vi "CSM - Send Message and Wait for Reply.vi"(6 "Response Timeout(5000ms)":i32=5000, 7 "Current Module(\"\" to generate a ID)":string, 8 "Error In (no error)":errorcluster, 9 "Target Module":string="Target", 10 "Arguments (\"\")":string, 11 "State":string="API State") -> (0 "error out":errorcluster, 2 "Response":string="DoA", 4 ">> Source CSM >>":string)   [LabVIEW 2020, in "Communicable State Machine.lvlib"]
doc: "Send a message to CSM specified and wait for the reply with timeout.\n\n<b>Inputs:</b>\n - <b>Target Module</b>: Target CSM Module name.\n - <b>State</b>: Message to send\n - <b>Arguments (\"\")</b>: Argument of the message.\n - <b>Response Timeout(5000ms)</b>: Timeout for waiting the response.\n - <b>Error In (no error)</b>: Error cluster\n\n<b>Outputs:</b>\n - <b>Arguments</b>: Response returned.\n - <b>error out</b>: Error cluster"
uses:
  Communicable State Machine.lvlib
  Priority Queue.lvclass/Priority Queue.ctl
  _CSMObj-Message Check.vi
  _CSMObj-Enqueue Cross-Module Message.vi
  _CSMOFGV Get.vi
  Enqueue Element.vi
  _CSMOFGV.vi
  CSM Not Allowed Message.vi
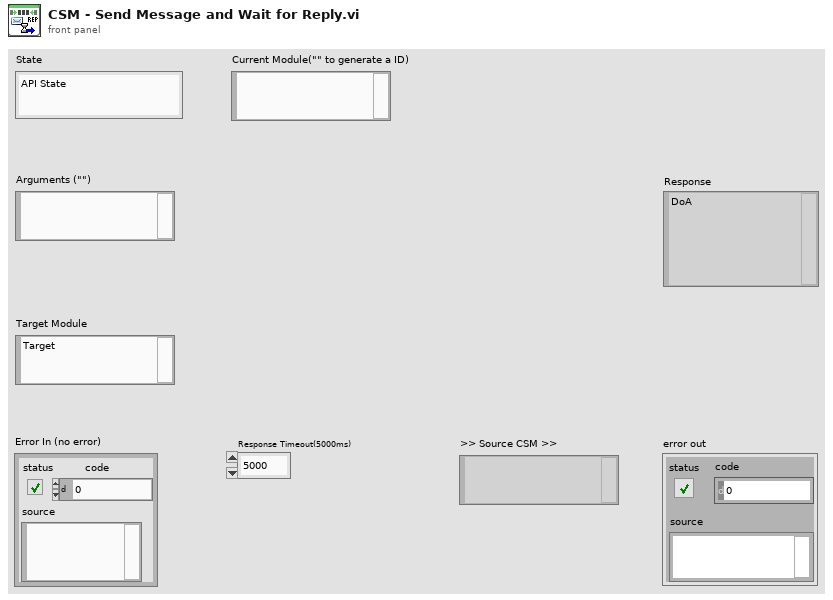
[diagram p1: front panel]
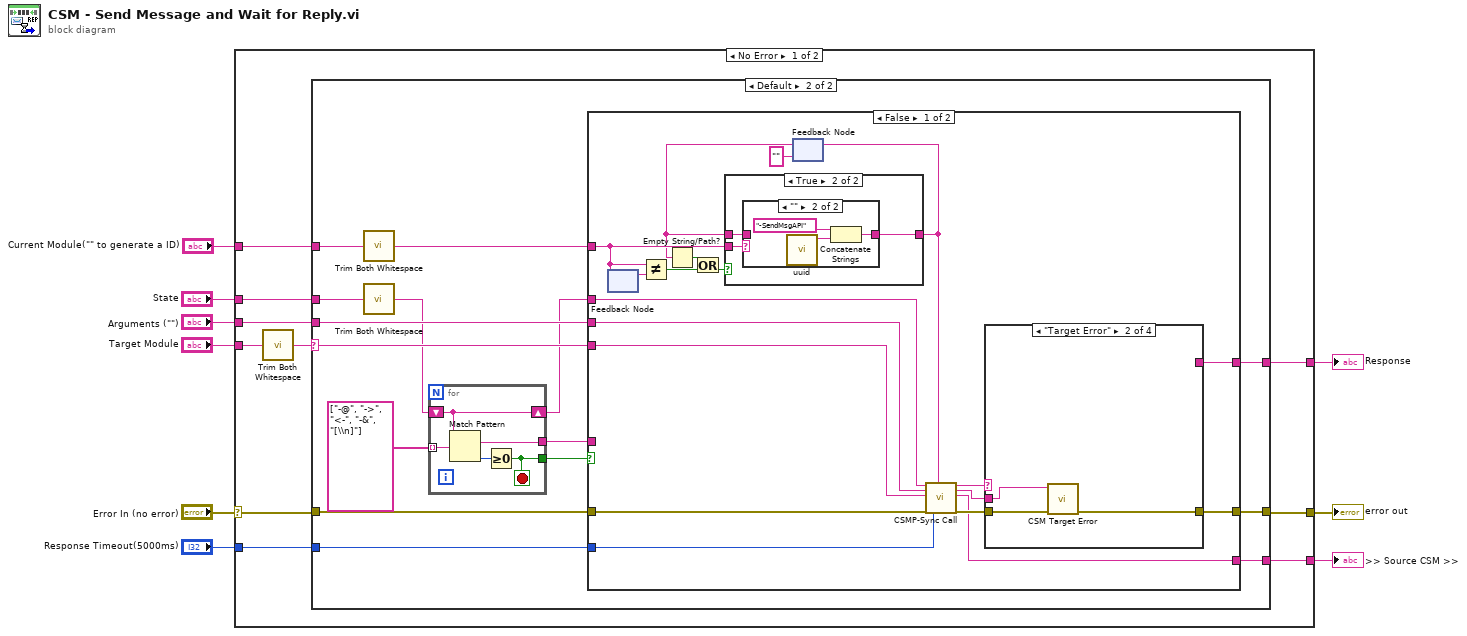
[diagram p0: block diagram]
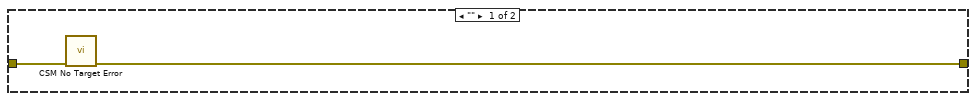
[diagram p2: hidden frame]
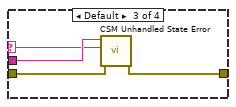
[diagram p6: hidden frame]
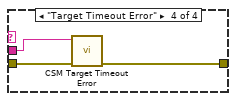
[diagram p7: hidden frame]
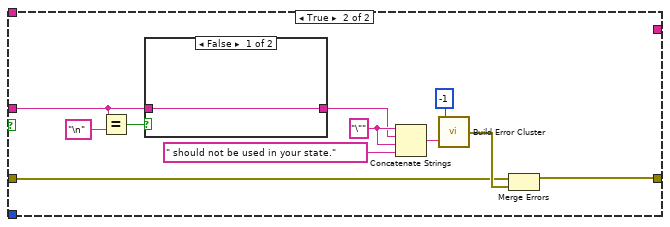
[diagram p8: hidden frame]
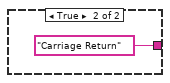
[diagram p9: hidden frame]
diagram:
  n1 = case shown="No Error" "Error In (no error)" {
    selector: "Error In (no error)" -> [w18 w94]
    tunnel: "State" -> [w19 _]
    tunnel: "Response Timeout(5000ms)" -> [w17 _]
    tunnel: [w13 w94] -> w6
    tunnel: [w16 _] -> w5
    tunnel: "Target Module" -> [w15 _]
    tunnel: "Arguments (\"\")" -> [w14 _]
    tunnel: "Current Module(\"\" to generate a ID)" -> [w11 _]
    tunnel: [w10 _] -> w1
    frame No Error {
      n2 = call "Trim Both Whitespace.vi"("string"=w15) -> ("trimmed string"=w12:string)  [unwired: 1 in]
      n3 = case shown="Default" w12 {
        selector: w12 -> [_ w33]
        tunnel: w18 -> [w21 w36]
        tunnel: w17 -> [_ w35]
        tunnel: [_ w34] -> w16
        tunnel: w14 -> [_ w32]
        tunnel: [w20 w31] -> w13
        tunnel: w19 -> [_ w30]
        tunnel: w11 -> [_ w23]
        tunnel: [_ w25] -> w10
        frame "" {
          n4 = call "CSM No Target Error.vi"("error in (no error)"=w21) -> ("error out"=w20:errorcluster)  [unwired: 10 in]
        }
        frame Default {
          n5 = call "Trim Both Whitespace.vi"("string"=w23) -> ("trimmed string"=w22:string)  [unwired: 1 in]
          n6 = call "Trim Both Whitespace.vi"("string"=w30) -> ("trimmed string"=w24:string)  [unwired: 1 in]
          n7 = for {
            shift-right: [w93] -> w29
            shift-left: w24 -> [w93]
            tunnel: string[] ["-@", "->", "<-", "-&", "[\\n]"] -> [w92] mode=indexing
            tunnel: [w90] -> w27
            tunnel: [w89] -> w28
            stop <- w89 stop-if-true
            n8 = Match Pattern(string=w93, regular expression=w92) -> (match substring=w90:string, offset past match=w91:i32)  [unwired: 1 in, 2 out]
            n9 = Greater Or Equal To 0?(x=w91) -> (x >= 0?=w89:bool)
          }
          n10 = case shown="False" w28 {
            tunnel: w36 -> [w55 w82]
            tunnel: w35 -> [w51 _]
            tunnel: [w46 _] -> w34
            tunnel: w33 -> [w52 _]
            tunnel: w32 -> [w53 _]
            tunnel: [w48 w83] -> w31
            tunnel: w29 -> [w54 _]
            tunnel: w27 -> [_ w78]
            tunnel: w22 -> [w42 _]
            tunnel: [w45 _] -> w25
            frame False {
              n11 = feedback-in #1(w42) -> ()
              n12 = feedback #1() -> (w43:string)  [unwired: 1 in]
              n13 = Not Equal?(x=w42, y=w43) -> (x != y?=w41:bool)
              n14 = feedback #2("") -> (w38:string)
              n15 = Empty String/Path?(string/path=w38) -> (empty?=w37:bool)
              n16 = Or(x=w37, y=w41) -> (x .or. y?=w39:bool)
              n17 = case shown="True" w39 {
                tunnel: w38 -> [w56 w59]
                tunnel: w42 -> [_ w58]
                tunnel: [w56 w57] -> w44
                frame False {
                }
                frame True {
                  n18 = case shown="\"\"" w58 {
                    selector: w58 -> [w60 _]
                    tunnel: [w60 w61] -> w57
                    tunnel: w59 -> [_ _]
                    frame Default {
                    }
                    frame "" {
                      n19 = call "uuid.vi"() -> ("UUID"=w62:string)  [unwired: 11 in]
                      n20 = Concatenate Strings("-SendMsgAPI" ("Name(\"\" to use uuid)"), w62) -> (w61:string)
                    }
                  }
                }
              }
              n21 = feedback-in #2(w44) -> ()
              n22 = call "CSMP-Sync Call.vi"("state"=w54, "args"=w53, "source/target"=w52, "Error in"=w55, "Response Timeout(5000ms)"=w51, "Module Name"=w44) -> ("state out"=w50:string, "args out"=w47:string, "source/target out"=w45:string, "error"=w49:errorcluster)  [unwired: 8 in, 2 out]
              n23 = case shown="\"Target Error\"" w50 {
                selector: w50 -> [_ _ w69 _]
                tunnel: w49 -> [w65 w67 w71 w74]
                tunnel: [w65 w66 w70 w73] -> w48
                tunnel: w47 -> [w64 w68 w72 w75]
                tunnel: [w64 _ _ _] -> w46
                frame "Response" {
                }
                frame "Target Error" {
                  n24 = call "CSM Target Error.vi"("error in (no error)"=w67, "Arguments(as CSM Name)"=w68) -> ("error out"=w66:errorcluster)  [unwired: 9 in]
                }
                frame Default {
                  n25 = call "CSM Unhandled State Error.vi"("error in (no error)"=w71, "Current State"=w69, "CSM Name"=w72) -> ("error out"=w70:errorcluster)  [unwired: 8 in]
                }
                frame "Target Timeout Error" {
                  n26 = call "CSM Target Timeout Error.vi"("error in (no error)"=w74, "Arguments(as CSM Name)"=w75) -> ("error out"=w73:errorcluster)  [unwired: 9 in]
                }
              }
            }
            frame True {
              w80 = "\"" ("string")
              n27 = Equal?(x=w78, y="\n" ("regular expression")) -> (x = y?=w76:bool)
              n28 = case shown="False" w76 {
                tunnel: [w87 "Carriage Return" ("State")] -> w79
                tunnel: w78 -> [w87 _]
                frame False {
                }
                frame True {
                }
              }
              n29 = Concatenate Strings(w80, w79, w80, " should not be used in your state." ("String to Prepend to source (\"\")")) -> (w81:string)
              n30 = call "Build Error Cluster.vi"("String to Prepend to source (\"\")"=w81, "code"=-1) -> ("error out"=w84:errorcluster)
              n31 = Merge Errors(w82, w84) -> (w83:errorcluster)
            }
          }
        }
      }
    }
    frame Error {
    }
  }
  "error out" <- w6
  "Response" <- w5
  ">> Source CSM >>" <- w1
